vi "array calculations.vi"() -> ()   [LabVIEW 2020]
panel:
  out "x-y":dbl[](array[numeric])
  out "y":dbl[](array[numeric])
  out "input array":dbl[](array[numeric])
  in  "new element":dbl
  out "x":dbl[](array[numeric])
  out "1array":dbl[](array[numeric])
  out "2d array":dbl[][](array[numeric])
  out "size(s)":i32
  out "new array":dbl[](array[numeric])
  in  "new element":i32
  in  "stop":bool
  in  "index":i32
  out "Array 2":dbl[](array[numeric])
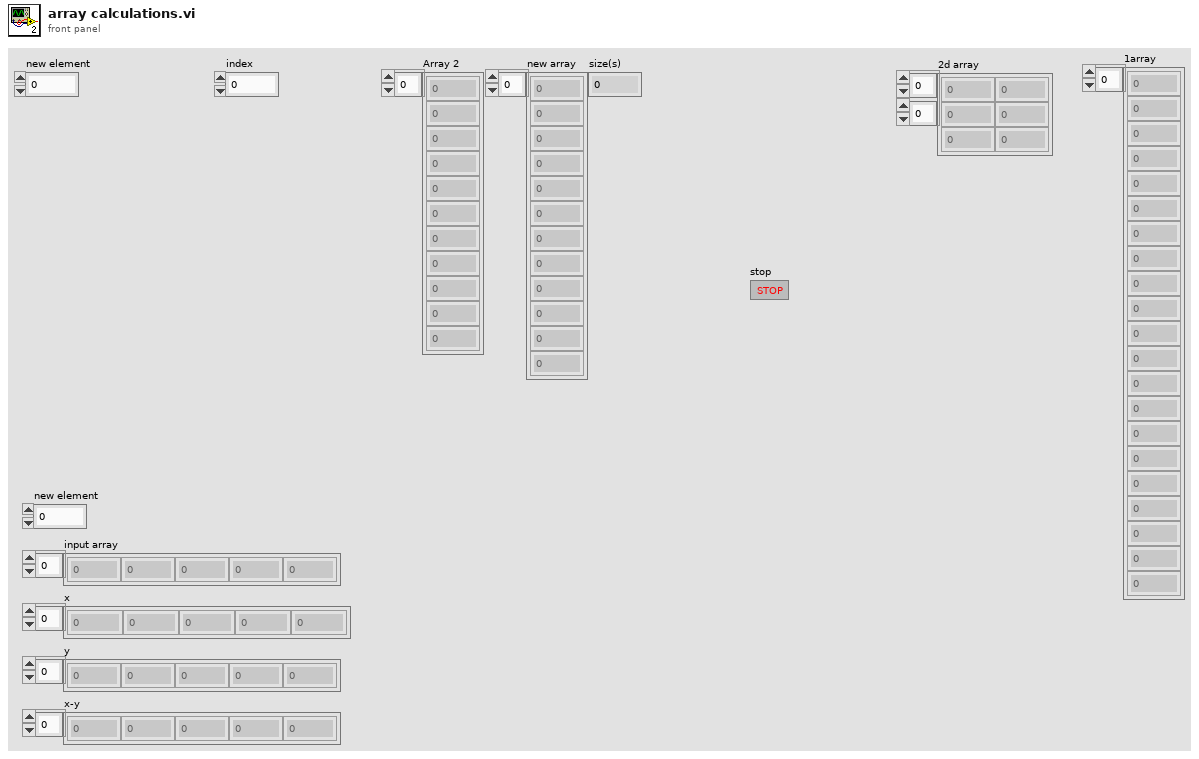
[diagram p1: front panel]
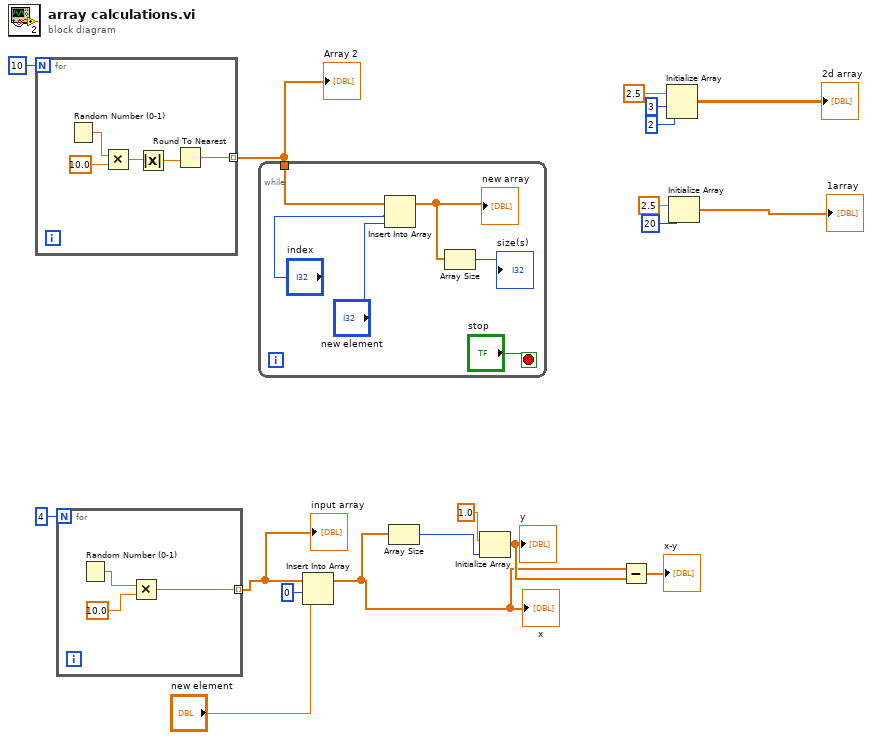
[diagram p0: block diagram]
diagram:
  n1 = for {
    N: 10 -> [_]
    tunnel: [w19] -> w17 mode=indexing
    n2 = Random Number (0-1)() -> (number: 0 to 1=w23:dbl)
    n3 = Multiply(x=w23, y=10.0) -> (x*y=w21:dbl)
    n4 = Absolute Value(x=w21) -> (abs(x)=w20:dbl)
    n5 = Round To Nearest(number=w20) -> (nearest integer value=w19:dbl)
  }
  "Array 2" <- w17
  n6 = for {
    N: 4 -> [_]
    tunnel: [w24] -> w6 mode=indexing
    n7 = Random Number (0-1)() -> (number: 0 to 1=w25:dbl)
    n8 = Multiply(x=w25, y=10.0) -> (x*y=w24:dbl)
  }
  "input array" <- w6
  n9 = while {
    tunnel: w17 -> [w31]
    stop <- "stop" stop-if-true
    n10 = Insert Into Array(array=w31, index="index", new element="new element") -> (w28:dbl[])
    "new array" <- w28
    n11 = Array Size(array=w28) -> (size(s)=→"size(s)":i32)
  }
  n12 = Insert Into Array(array=w6, index=0, new element="new element") -> (w1:dbl[])
  "x" <- w1
  n13 = Array Size(array=w1) -> (size(s)=w5:i32)
  n14 = Initialize Array(1.0 ("element"), w5) -> (w2:dbl[])
  "y" <- w2
  n15 = Subtract(x=w1, y=w2) -> (x-y=→"x-y":dbl[])
  n16 = Initialize Array(2.5 ("element"), 3 ("dimension size"), 2 ("dimension size")) -> (→"2d array":dbl[][])
  n17 = Initialize Array(2.5 ("element"), 20 ("dimension size")) -> (→"1array":dbl[])
